vi "Read TLS.vi"(8 "error in":errorcluster, 11 "Serial in":refnum<class "MB_Master_Serial.lvclass">[](array[class])) -> (0 "error out":errorcluster, 3 "Serial out":refnum<class "MB_Master_Serial.lvclass">[](array[class]))   [LabVIEW 2017, in "Akwizycja.lvlib"]
uses:
  Akwizycja.lvlib
  <vilib>/Plasmionique/MB Master/MB_Master_Serial/MB_Master_Serial.lvclass
  D:/Program Files (x86)/National Instruments/LabVIEW 2017/vi.lib/Plasmionique/MB Master/MB_Master/MB_Master.lvclass
  <vilib>/Plasmionique/MB Master/MB Master.lvlib
panel:
  in  "TLS Cluster":T1
  in  "TLS cluster":T1
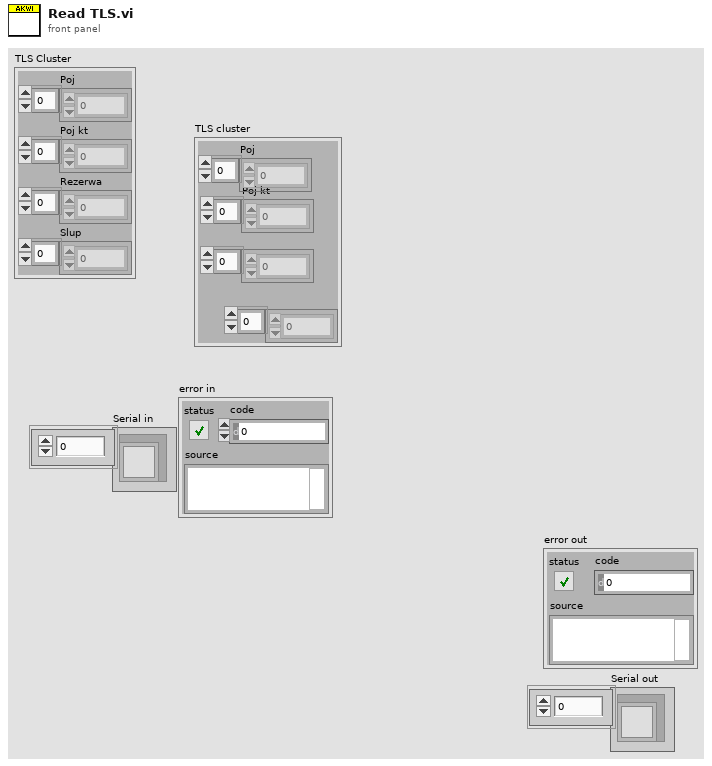
[diagram p1: front panel]
types:
  T1 = cluster{"Poj":sgl[], "Poj kt":sgl[], "Rezerwa":sgl[], "Slup":sgl[]}
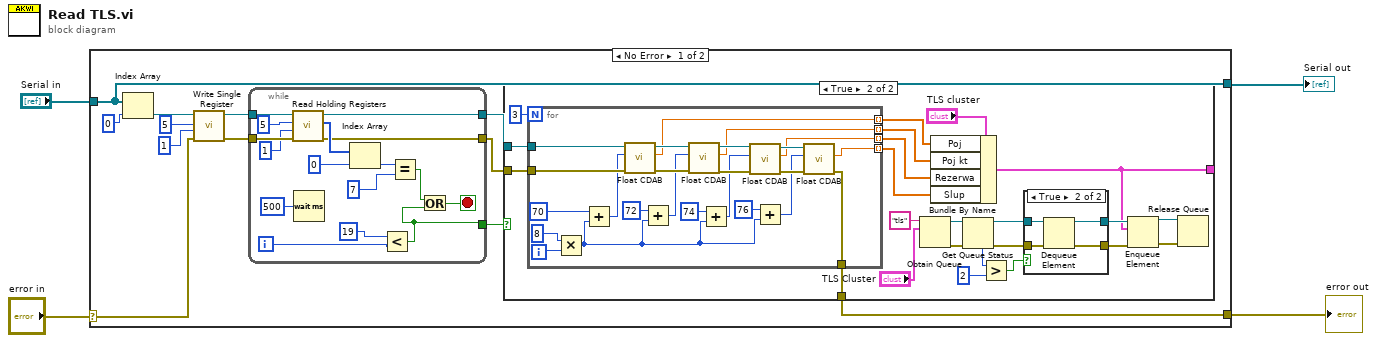
[diagram p0: block diagram]
diagram:
  n1 = case shown="No Error" "error in" {
    selector: "error in" -> [w12 w88]
    tunnel: [w5 w88] -> w3
    tunnel: "Serial in" -> [w11 w87]
    tunnel: [w11 w87] -> w1
    frame No Error {
      n2 = Index Array(array=w11, index=0) -> (element=w15:refnum<class "MB_Master_Serial.lvclass">)
      n3 = call <vilib>:"Write Single Register.vi"("error in (no error)"=w12, "value"=u16 1, "address"=u16 5 ("starting address"), "MB session in"=w15) -> ("error out"=w9:errorcluster, "MB session out"=w10:refnum<class "MB_Master_Serial.lvclass">)  [unwired: 6 in]
      n4 = while {
        tunnel: w10 -> [w85]
        tunnel: w9 -> [w84]
        tunnel: [w71] -> w8
        tunnel: [w75] -> w7
        tunnel: [w74] -> w6
        i -> [w72]
        stop <- w76 stop-if-true
        n5 = call <vilib>:"Read Holding Registers.vi"("error in (no error)"=w84, "quantity"=u16 1, "starting address"=u16 5, "MB session in"=w85) -> ("error out"=w75:errorcluster, "Registers"=w79:u16[], "MB session out"=w74:refnum<class "MB_Master_Serial.lvclass">)  [unwired: 5 in]
        n6 = Wait (ms)(milliseconds to wait=u32 500) -> ()  [unwired: 1 out]
        n7 = Index Array(array=w79, index=0) -> (element=w78:u16)
        n8 = Less?(x=19, y=w72) -> (x < y?=w71:bool)
        n9 = Equal?(x=w78, y=u16 7 ("quantity")) -> (x = y?=w77:bool)
        n10 = Or(x=w77, y=w71) -> (x .or. y?=w76:bool)
      }
      n11 = case shown="True" w8 {
        tunnel: w7 -> [w17 w39]
        tunnel: w6 -> [_ w40]
        tunnel: [_ w20] -> _
        tunnel: [w17 w32] -> w5
        frame False {
        }
        frame True {
          n12 = for {
            N: 3 -> [_]
            tunnel: w40 -> [w70]
            tunnel: w39 -> [w69]
            tunnel: [w51] -> w36 mode=indexing
            tunnel: [w50] -> w35 mode=indexing
            tunnel: [w49] -> w34 mode=indexing
            tunnel: [w48] -> w33 mode=indexing
            tunnel: [w47] -> w32
            i -> [w64]
            n13 = Multiply(x=8, y=w64) -> (x*y=w59:i32)
            n14 = Add(x=u16 70 ("starting address"), y=w59) -> (x+y=w65:i32)
            n15 = call "Float CDAB.vi"("error in"=w69, "starting address"=w65, "Serial in"=w70) -> ("error out"=w68:errorcluster, "ABCD"=w51:sgl, "Serial out"=w67:refnum<class "MB_Master_Serial.lvclass">)  [unwired: 6 in]
            n16 = Add(x=72, y=w59) -> (x+y=w58:i32)
            n17 = call "Float CDAB.vi"("error in"=w68, "starting address"=w58, "Serial in"=w67) -> ("error out"=w57:errorcluster, "ABCD"=w50:sgl, "Serial out"=w56:refnum<class "MB_Master_Serial.lvclass">)  [unwired: 6 in]
            n18 = Add(x=74, y=w59) -> (x+y=w55:i32)
            n19 = call "Float CDAB.vi"("error in"=w57, "starting address"=w55, "Serial in"=w56) -> ("error out"=w54:errorcluster, "ABCD"=w49:sgl, "Serial out"=w53:refnum<class "MB_Master_Serial.lvclass">)  [unwired: 6 in]
            n20 = Add(x=76, y=w59) -> (x+y=w52:i32)
            n21 = call "Float CDAB.vi"("error in"=w54, "starting address"=w52, "Serial in"=w53) -> ("error out"=w47:errorcluster, "ABCD"=w48:sgl)  [unwired: 6 in, 1 out]
          }
          n22 = Obtain Queue(name (unnamed)="tls", element data type="TLS Cluster") -> (queue out=w22:refnum<queue>, error out=w21:errorcluster)  [unwired: 3 in, 1 out]
          n23 = Bundle By Name(cluster="TLS cluster", "Poj"=w36, "Poj kt"=w35, "Rezerwa"=w34, "Slup"=w33) -> (w20:T1)
          n24 = Get Queue Status(queue=w22, error in (no error)=w21) -> (queue out=w26:refnum<queue>, error out=w29:errorcluster, # elements in queue=w28:i32)  [unwired: 1 in, 5 out]
          n25 = Greater?(x=w28, y=2) -> (0:w25:bool)
          n26 = case shown="True" w25 {
            tunnel: w29 -> [w41 w46]
            tunnel: w26 -> [w42 w45]
            tunnel: [w42 w44] -> w24
            tunnel: [w41 w43] -> w23
            frame False {
            }
            frame True {
              n27 = Dequeue Element(queue=w45, error in (no error)=w46) -> (queue out=w44:refnum<queue>, error out=w43:errorcluster)  [unwired: 1 in, 2 out]
            }
          }
          n28 = Enqueue Element(queue=w24, element=w20, error in (no error)=w23) -> (queue out=w31:refnum<queue>, error out=w30:errorcluster)  [unwired: 1 in, 1 out]
          n29 = Release Queue(queue=w31, error in (no error)=w30) -> ()  [unwired: 1 in, 3 out]
        }
      }
    }
    frame Error {
    }
  }
  "error out" <- w3
  "Serial out" <- w1
